vi "Write Shared Event References.vi"(8 "error in (no error)":errorcluster, 10 "Shared Event References":T1, 11 "UDP_Service in":refnum<class "UDP_Service.lvclass">) -> (0 "error out":errorcluster, 3 "UDP_Service out":refnum<class "UDP_Service.lvclass">)   [LabVIEW 2016, in "CoreAssertAPI.lvlib" / "UDP_Service.lvclass"]
uses:
  UDP_Service.lvclass
  External Display/Shared Event References.ctl
  Assert Packet.ctl
  Message Data.ctl
  VI References.ctl
  Classes/Filters/Base Filter.lvclass
  UDP_Service.lvclass/UDP_Service.ctl
  CoreAssertAPI.lvlib
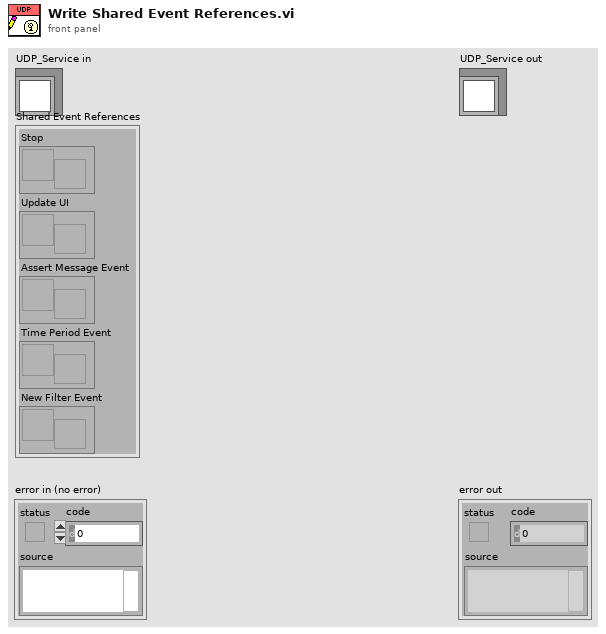
[diagram p1: front panel]
types:
  T1 = typedef "CoreAssertAPI.lvlib/Shared Event References.ctl" = cluster{"Stop":refnum<user-event>, "Update UI":refnum<user-event>, "Assert Message Event":refnum<user-event>, "Time Period Event":refnum<user-event>, "New Filter Event":refnum<user-event>}
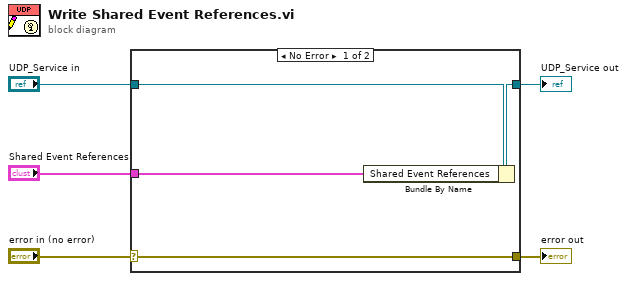
[diagram p0: block diagram]
diagram:
  n1 = case shown="No Error" "error in (no error)" {
    selector: "error in (no error)" -> [w9 w10]
    tunnel: [w9 w10] -> w4
    tunnel: [w7 w11] -> w2
    tunnel: "UDP_Service in" -> [w8 w11]
    tunnel: "Shared Event References" -> [w6 _]
    frame No Error {
      n2 = Bundle By Name(cluster=w8, "Shared Event References"=w6) -> (w7:refnum<class "UDP_Service.lvclass">)
    }
    frame Error {
    }
  }
  "error out" <- w4
  "UDP_Service out" <- w2
